vi "TPISend.vi"(8 "error in (no error)":errorcluster, 9 "Read Responce":bool, 10 "write buffer":string, 11 "VISA resource name":refnum<visa-resource-name>) -> (0 "error out":errorcluster, 2 "Hex Responce":string, 3 "VISA resource name out":refnum<visa-resource-name>)   [LabVIEW 2019]
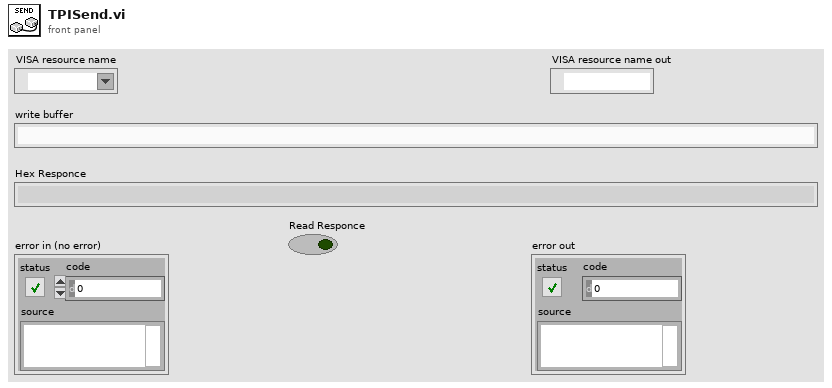
[diagram p1: front panel]
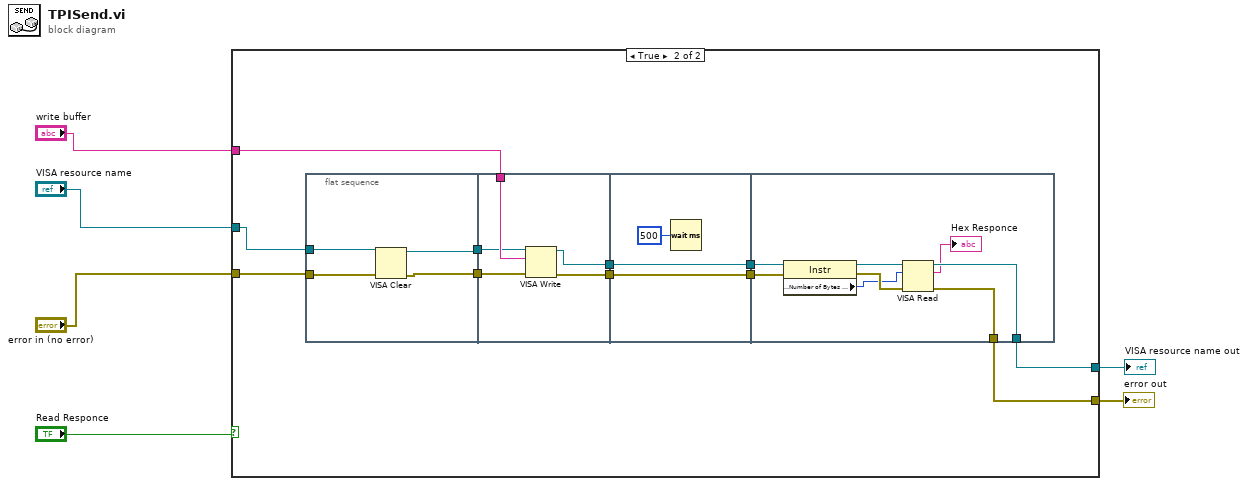
[diagram p0: block diagram]
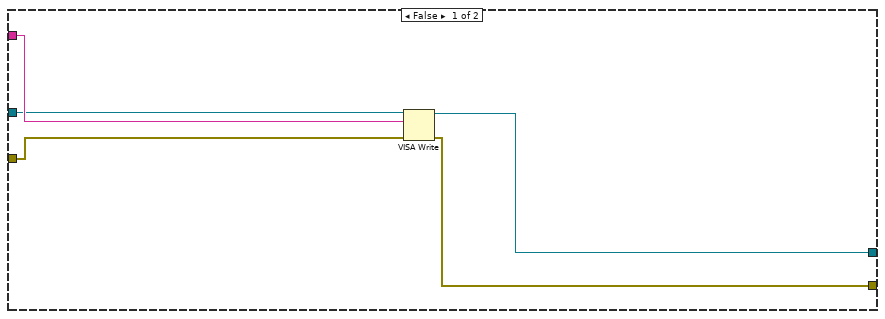
[diagram p2: hidden frame]
diagram:
  n1 = case shown="True" "Read Responce" {
    tunnel: [w7 w18] -> w6
    tunnel: [w8 w17] -> w5
    tunnel: "VISA resource name" -> [w9 w15]
    tunnel: "write buffer" -> [w10 w14]
    tunnel: "error in (no error)" -> [w11 w16]
    frame False {
      n2 = VISA Write(VISA resource name=w9, write buffer=w10, error in (no error)=w11) -> (VISA resource name out=w8:refnum<visa-resource-name>, error out=w7:errorcluster)  [unwired: 1 out]
    }
    frame True {
      n3 = flat-sequence {
        tunnel: w16 -> [w25]
        tunnel: w15 -> [w26]
        tunnel: [w24] -> w13
        tunnel: [w23] -> w12
        tunnel: [w31] -> w22
        tunnel: [w30] -> w21
        tunnel: w14 -> [w29]
        tunnel: w13 -> [w28]
        tunnel: w12 -> [w27]
        tunnel: [w34] -> w20
        tunnel: w22 -> [w34]
        tunnel: [w33] -> w19
        tunnel: w21 -> [w33]
        tunnel: w20 -> [w39]
        tunnel: w19 -> [w38]
        tunnel: [w37] -> w18
        tunnel: [w36] -> w17
        frame #0 {
          n4 = VISA Clear(VISA resource name=w26, error in (no error)=w25) -> (VISA resource name out=w24:refnum<visa-resource-name>, error out=w23:errorcluster)
        }
        frame #1 {
          n5 = VISA Write(VISA resource name=w28, write buffer=w29, error in (no error)=w27) -> (VISA resource name out=w30:refnum<visa-resource-name>, error out=w31:errorcluster)  [unwired: 1 out]
        }
        frame #2 {
          n6 = Wait (ms)(milliseconds to wait=u32 500) -> ()  [unwired: 1 out]
        }
        frame #3 {
          n7 = property class="Instr"(reference=w38, error in=w39) -> (reference out=w41:refnum<visa-resource-name>, error out=w42:errorcluster, "Serial Settings:Number of Bytes at Serial Port"=w40:u32)
          n8 = VISA Read(VISA resource name=w41, byte count=w40, error in (no error)=w42) -> (VISA resource name out=w36:refnum<visa-resource-name>, read buffer=→"Hex Responce":string, error out=w37:errorcluster)  [unwired: 1 out]
        }
      }
    }
  }
  "error out" <- w6
  "VISA resource name out" <- w5
